vi "Rotate Preview Map.vi"(8 "error in (no error)":errorcluster, 10 "Rotation Angle":dbl, 11 "Map Model in":refnum<class "Map Model.lvclass">) -> (0 "error out":errorcluster, 3 "Map Model out":refnum<class "Map Model.lvclass">)   [LabVIEW 2020, in "Map Model.lvlib" / "Map Model.lvclass"]
uses:
  Map Model.lvclass
  Map Model.lvclass/Map Model.ctl
  Tools/Tool/Tool.lvclass/Tool.ctl
  Tools/Tool/Tool.lvclass
panel:
  # "NOTICE -- YOU MUST LEAVE THIS NOTICE IN PLACE.\n\nCopyright (c) 2017, LIANG LIU Shawn.Liu.cn@gmail.com\nAll rights reserved.\n\nRedistribution and use in source and binary forms, with or without modification, are permitted provided that the following conditions are met:\n-Redistributions of source code must retain the above copyright notice, this list of conditions and the following disclaimer.\n-Redistributions in binary form must reproduce the above copyright notice, this list of conditions and the following disclaimer in the documentation and/or other materials provided with the distribution.\n-Neither the name of the eLp nor the names of its contributors may be used to endorse or promote products derived from this software without specific prior written permission.\n\nTHIS SOFTWARE IS PROVIDED BY THE COPYRIGHT HOLDERS AND CONTRIBUTORS \"AS IS\" AND ANY EXPRESS OR IMPLIED WARRANTIES, INCLUDING, BUT NOT LIMITED TO, THE IMPLIED WARRANTIES OF MERCHANTABILITY AND FITNESS FOR A PARTICULAR PURPOSE ARE DISCLAIMED. IN NO EVENT SHALL THE COPYRIGHT HOLDER OR CONTRIBUTORS BE LIABLE FOR ANY DIRECT, INDIRECT, INCIDENTAL, SPECIAL, EXEMPLARY, OR CONSEQUENTIAL DAMAGES (INCLUDING, BUT NOT LIMITED TO, PROCUREMENT OF SUBSTITUTE GOODS OR SERVICES; LOSS OF USE, DATA, OR PROFITS; OR BUSINESS INTERRUPTION) HOWEVER CAUSED AND ON ANY THEORY OF LIABILITY, WHETHER IN CONTRACT, STRICT LIABILITY, OR TORT (INCLUDING NEGLIGENCE OR OTHERWISE) ARISING IN ANY WAY OUT OF THE USE OF THIS SOFTWARE, EVEN IF ADVISED OF THE POSSIBILITY OF SUCH DAMAGE."
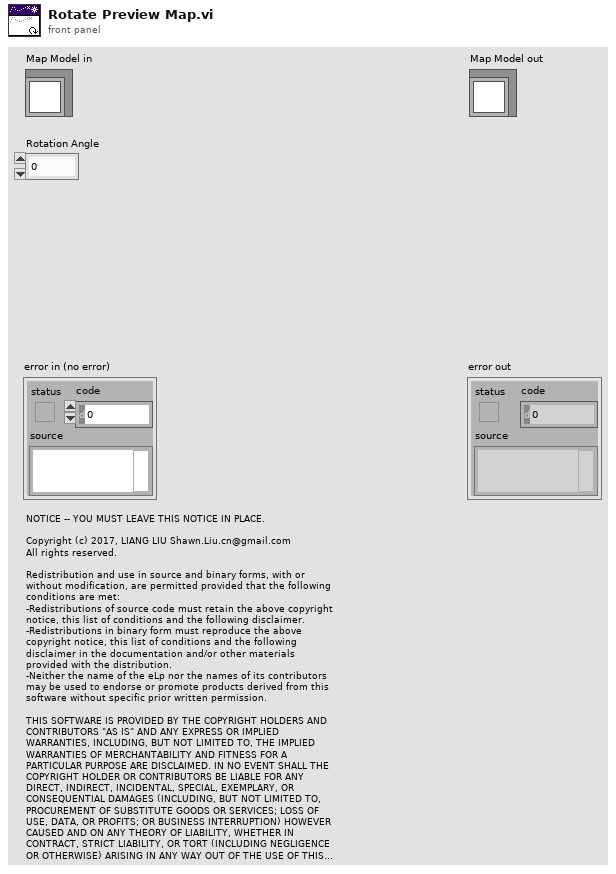
[diagram p1: front panel]
types:
  T1 = typedef "LVPoint32TypeDef.ctl" = cluster{"Horizontal":i32, "Vertical":i32}
  T2 = typedef "LVPointTypeDef.ctl" = cluster{"Horizontal":i16, "Vertical":i16}
  T3 = cluster{"Occupied Color":cluster{"Value":u8, "Color":u32}, "Free Color":cluster{"Value":u8, "Color":u32}, "Unknown Color":cluster{"Value":u8, "Color":u32}}
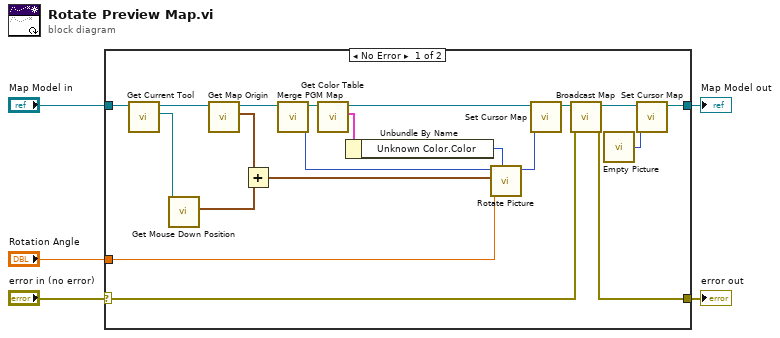
[diagram p0: block diagram]
diagram:
  n1 = case shown="No Error" "error in (no error)" {
    selector: "error in (no error)" -> [w22 w27]
    tunnel: "Map Model in" -> [w25 w26]
    tunnel: [w24 w26] -> w4
    tunnel: "Rotation Angle" -> [w23 _]
    tunnel: [w21 w27] -> w1
    frame No Error {
      n2 = call "Get Current Tool.vi"("Map Model in"=w25) -> ("Current Tool"=w17:refnum<class "Tool.lvclass">, "Map Model out"=w18:refnum<class "Map Model.lvclass">)  [unwired: 9 in]
      n3 = call "Get Mouse Down Position.vi"("Tool in"=w17) -> ("Mouse Down Position"=w9:T1)  [unwired: 9 in, 1 out]
      n4 = call "Get Map Origin.vi"("Map Model in"=w18) -> ("Map Origin"=w13:T2, "Map Model out"=w14:refnum<class "Map Model.lvclass">)  [unwired: 9 in]
      n5 = Add(x=w13, y=w9) -> (x+y=w11:T1)
      n6 = call "Merge PGM Map.vi"("Map Model in"=w14) -> ("Map"=w8:picture, "Map Model out"=w20:refnum<class "Map Model.lvclass">)  [unwired: 7 in, 2 out]
      n7 = call "Get Color Table.vi"("Map Model in"=w20) -> ("Color Table"=w15:T3, "Map Model out"=w16:refnum<class "Map Model.lvclass">)  [unwired: 9 in]
      n8 = Unbundle By Name(w15) -> ("Unknown Color.Color"=w10:u32)
      n9 = call "Rotate Picture.vi"("Unknown Color (black)"=w10, "Rotation Angle (degree)"=w23, "Center"=w11, "Picture in"=w8) -> ("Picture out"=w12:picture)  [unwired: 7 in]
      n10 = call "Set Cursor Map.vi"("Cursor Map"=w12, "Map Model in"=w16) -> ("Map Model out"=w6:refnum<class "Map Model.lvclass">)  [unwired: 9 in]
      n11 = call "Broadcast Map.vi"("error in (no error)"=w22, "Map Model in"=w6) -> ("error out"=w21:errorcluster, "Map Model out"=w19:refnum<class "Map Model.lvclass">)  [unwired: 8 in]
      n12 = call "Empty Picture"() -> ("empty picture"=w7:picture)
      n13 = call "Set Cursor Map.vi"("Cursor Map"=w7, "Map Model in"=w19) -> ("Map Model out"=w24:refnum<class "Map Model.lvclass">)  [unwired: 9 in]
    }
    frame Error {
    }
  }
  "error out" <- w1
  "Map Model out" <- w4
